vi "Old Washing Machine Analog Timer (Control + Indicator).vi"() -> ()   [LabVIEW 2016]
panel:
  in  "Dial":dbl(knob) scale=0.0..10.0
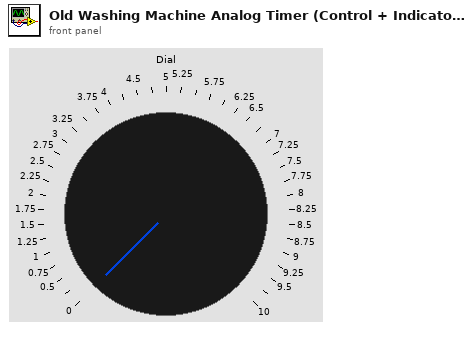
[diagram p1: front panel]
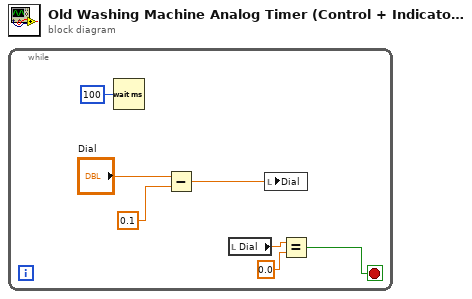
[diagram p0: block diagram]
diagram:
  n1 = while {
    stop <- w5 stop-if-true
    n2 = Wait (ms)(milliseconds to wait=u32 100) -> ()  [unwired: 1 out]
    n3 = Subtract(x="Dial", y=0.1 ("x")) -> (x-y=w7:dbl)
    n4 = local read "Dial"() -> (w6:dbl)
    n5 = local write "Dial"(w7) -> ()
    n6 = Equal?(x=w6, y=0.0) -> (x = y?=w5:bool)
  }
